vi "Monochromator API.vi"(7 "Comm":T3, 8 "error in (no error)":errorcluster, 11 "Data in out":T1={"MonoCr Port"="COM3", "Grating Selection"=enum."Grating@1", "Connection?"=TRUE, "LED Comm"=enum."LED@1", "Intensity Value"=0, "Grating Number"=1, "Wavenumber"=0, "Slit Width"=8, "Filter Num"=3, "Grating Density"=1200, "Wavelength(nm)"=400, "offset"=0.0}) -> (0 "error out":errorcluster, 2 "Connection?":bool, 3 "Data in out":T1)   [LabVIEW 2018]
uses:
  Controls/API Command.ctl
  Controls/Data highway.ctl
  Controls/LED intensity Command.ctl
  b728575c-1e5c-4404-af7d-9a6214211f88.vi
  1f586dfe-ed04-43a5-ae94-1c2b0e0186bb.vi
  98e89029-55c1-4bbe-a736-8af9f524e05c.vi
  8abd1e0c-5597-4431-9aed-95265bc6d135.vi
  59c60f5b-33d1-4c58-8755-e7aa3c9d5b29.vi
  a81fc492-f652-474c-8cd8-c09e6a443d99.vi
  8c89b708-3d56-4cfa-8980-e2557ccac631.vi
  0ff77aef-d465-45ef-9306-fcadcf69f8fd.vi
  4d5c323e-a406-4662-8192-a49ad5524d44.vi
  <vilib>/Instr/_visa.llb/VISA Configure Serial Port (Instr).vi
panel:
  in  "MonoCr Port":refnum<visa-resource-name>
  in  "Inc":bool
  out "error out":errorcluster
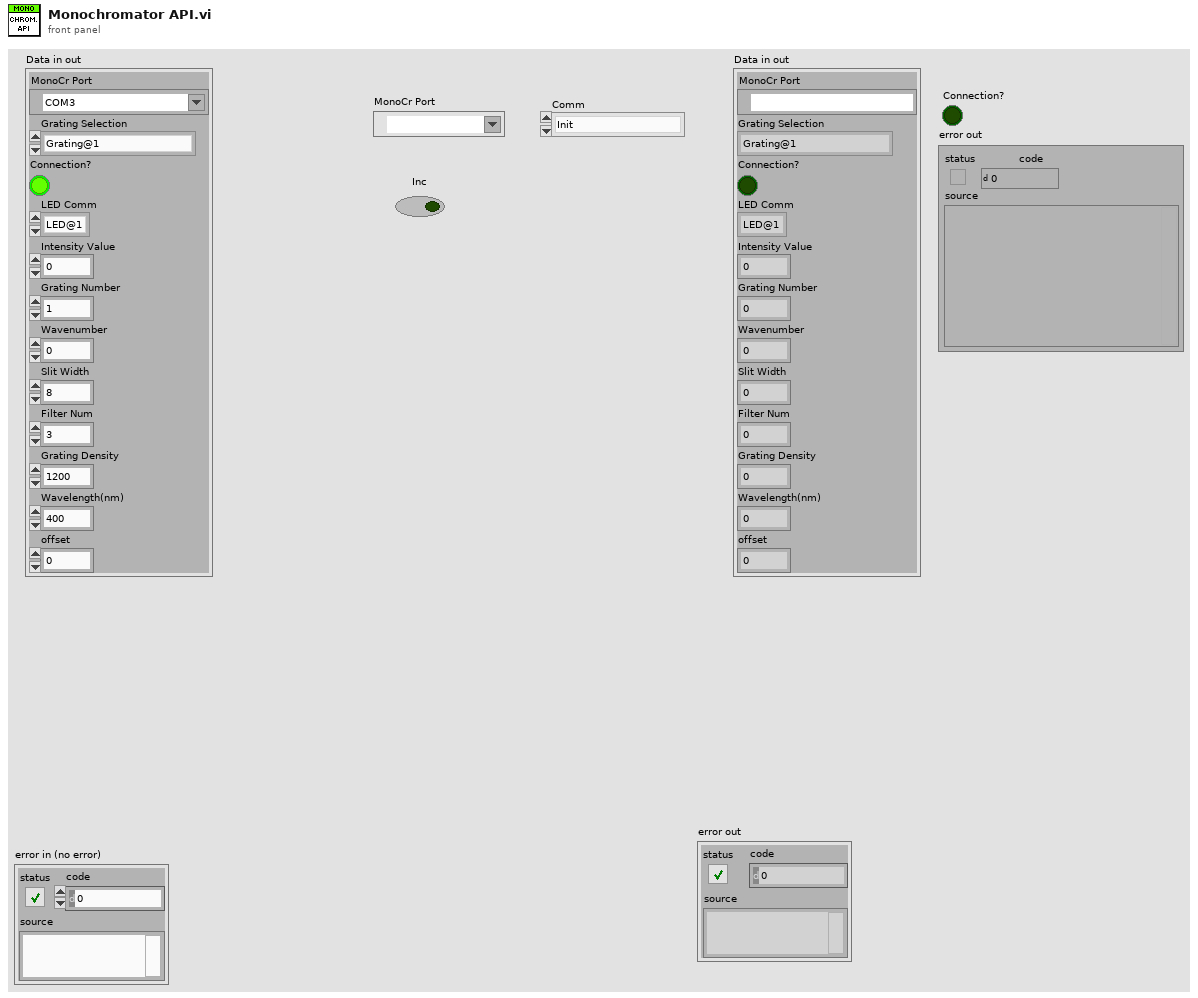
[diagram p1: front panel]
types:
  T1 = typedef "Data highway.ctl" = cluster{"MonoCr Port":refnum<visa-resource-name>, "Grating Selection":enum16{"Grating@1", "Grating@2"}, "Connection?":bool, "LED Comm":T2, "Intensity Value":i32, "Grating Number":i32, "Wavenumber":i32, "Slit Width":i32, "Filter Num":i32, "Grating Density":i32, "Wavelength(nm)":i32, "offset":dbl}
  T2 = typedef "LED intensity Command.ctl" = enum16{"LED@1", "LED@2"}
  T3 = typedef "API Command.ctl" = enum16{"Init", "Device Check", "Grating Density@1", "Grating Density@2", "SetWavelength", "Filter Selection", "Shutter open", "Shutter close", "LED Intensity", "Set Grating", "Slit Width", "Stop running", "Reset Mono", "Close"}
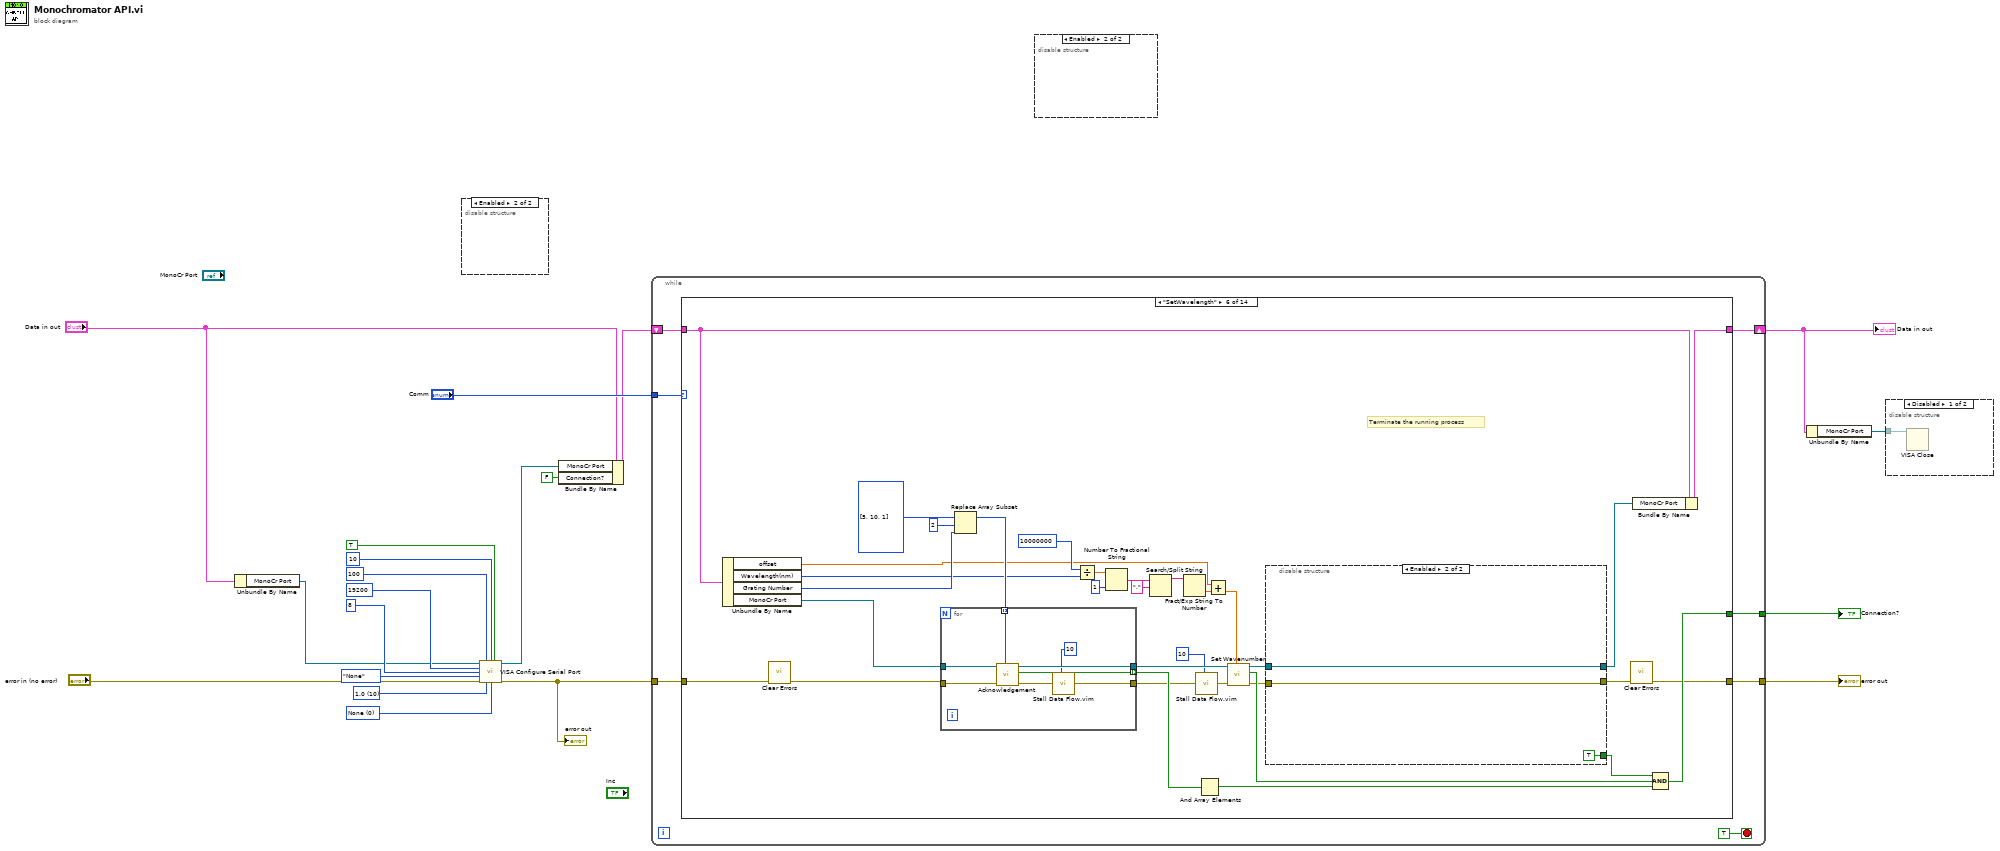
[diagram p0: block diagram]
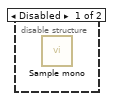
[diagram p3: hidden frame]
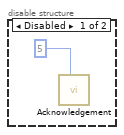
[diagram p4: hidden frame]
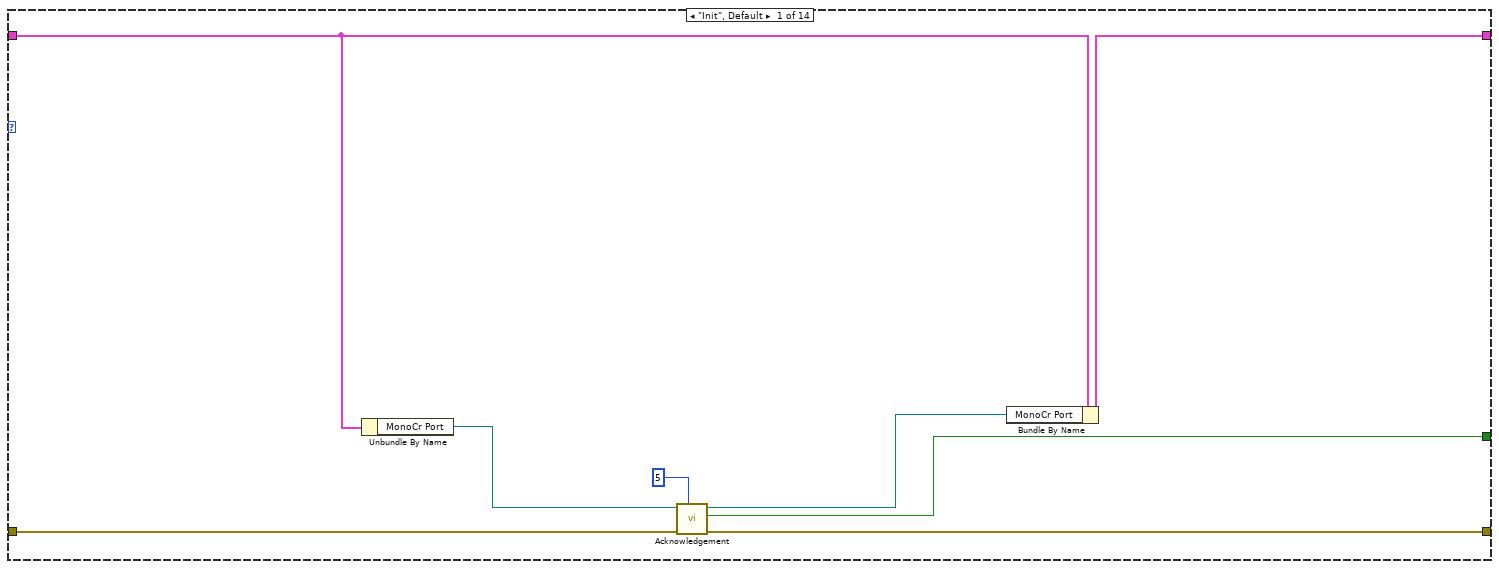
[diagram p5: hidden frame]
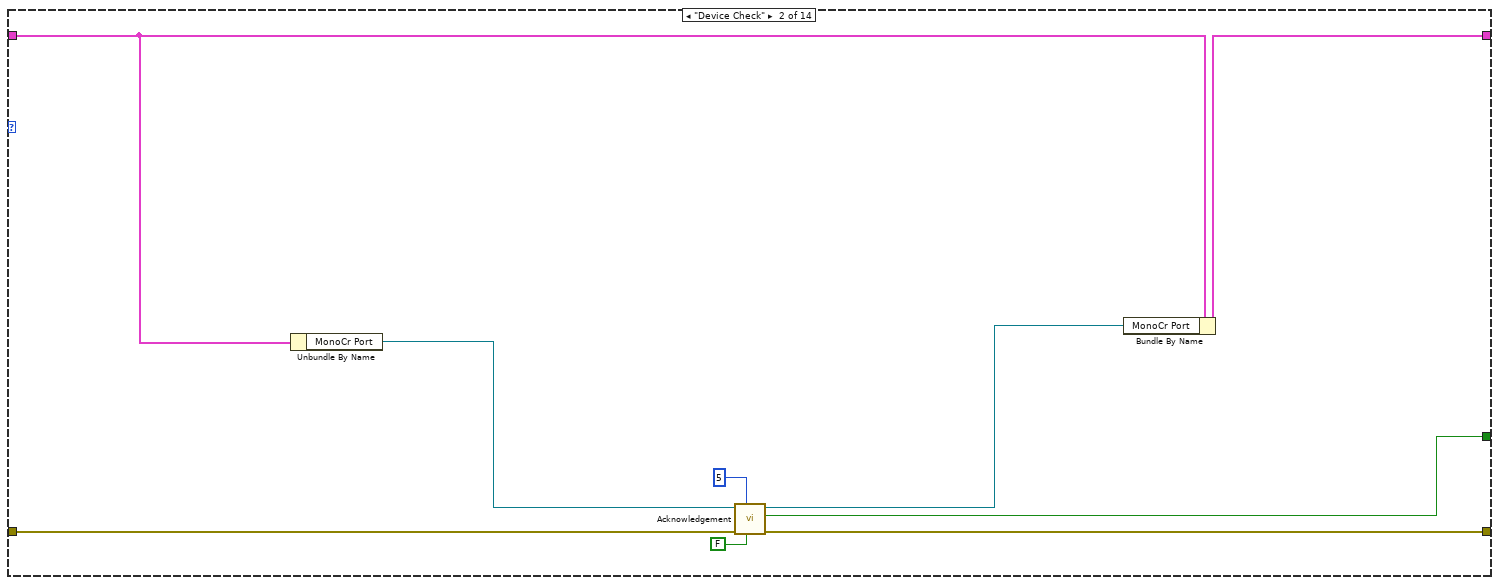
[diagram p6: hidden frame]
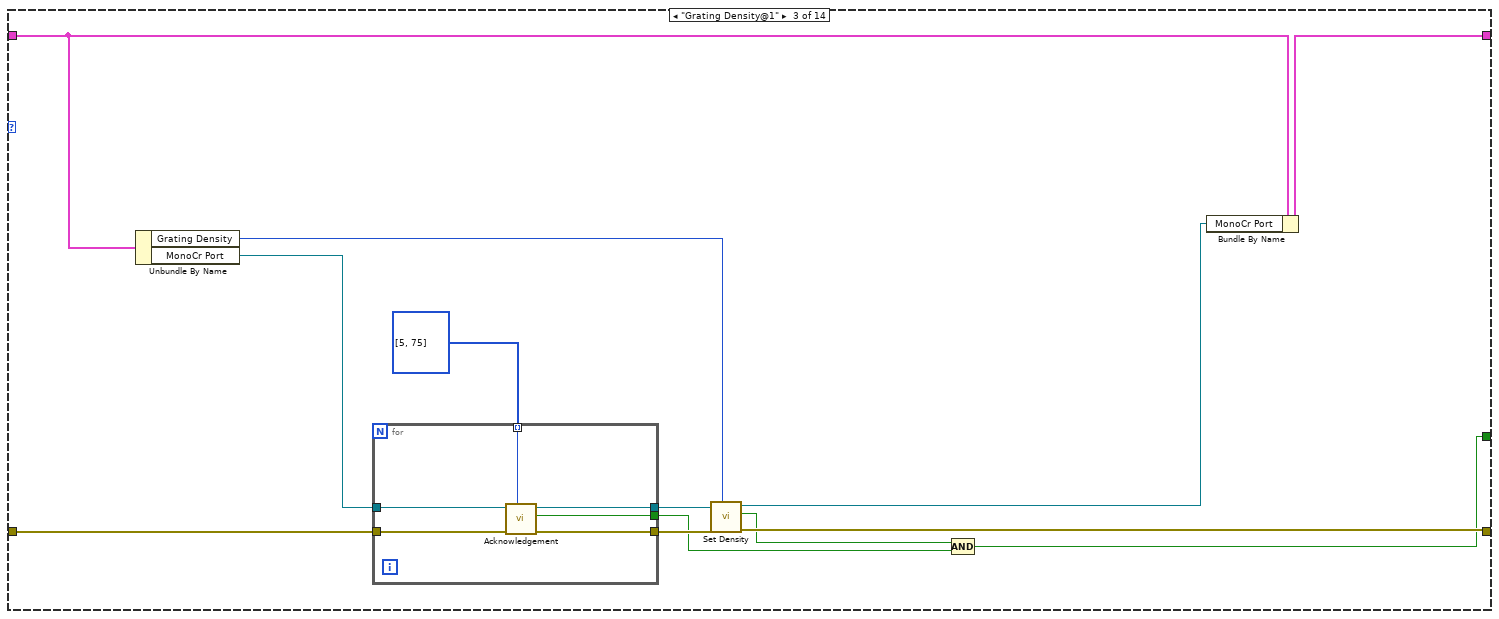
[diagram p7: hidden frame]
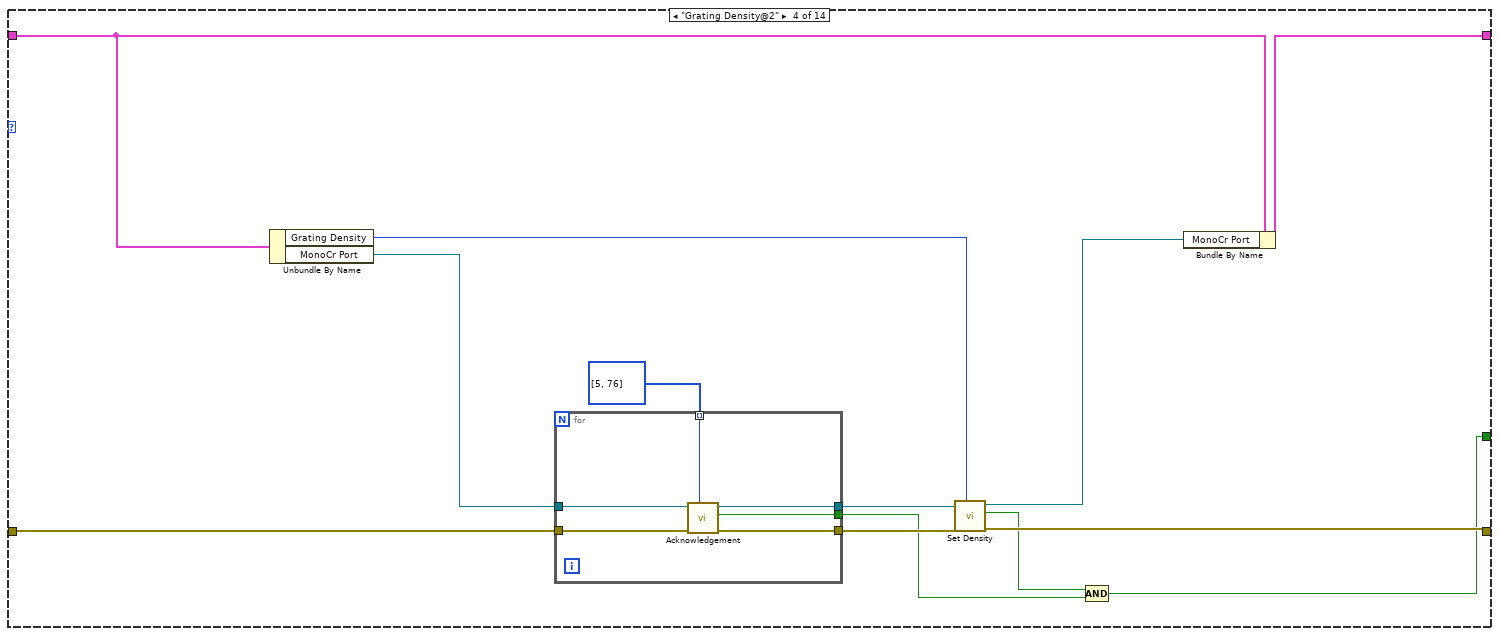
[diagram p8: hidden frame]
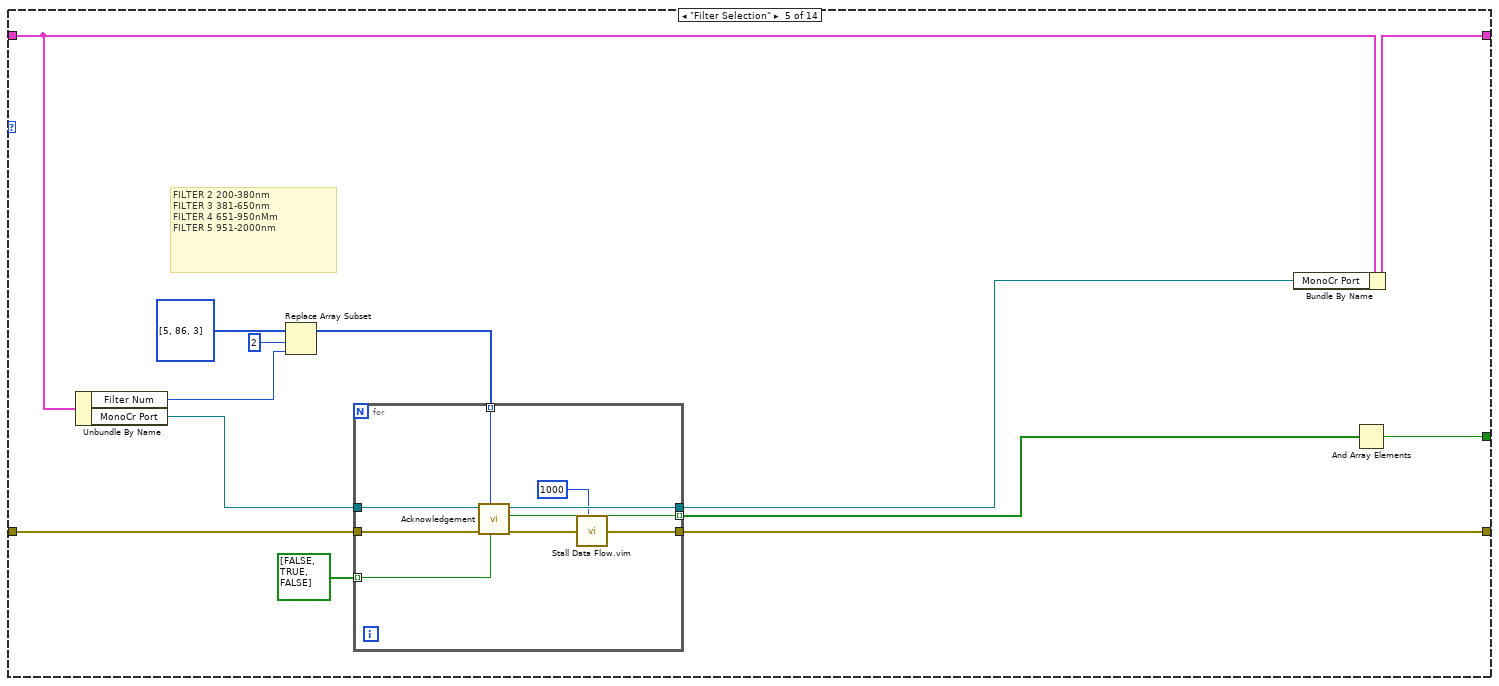
[diagram p9: hidden frame]
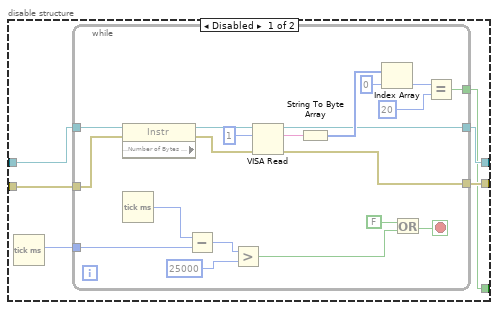
[diagram p10: hidden frame]
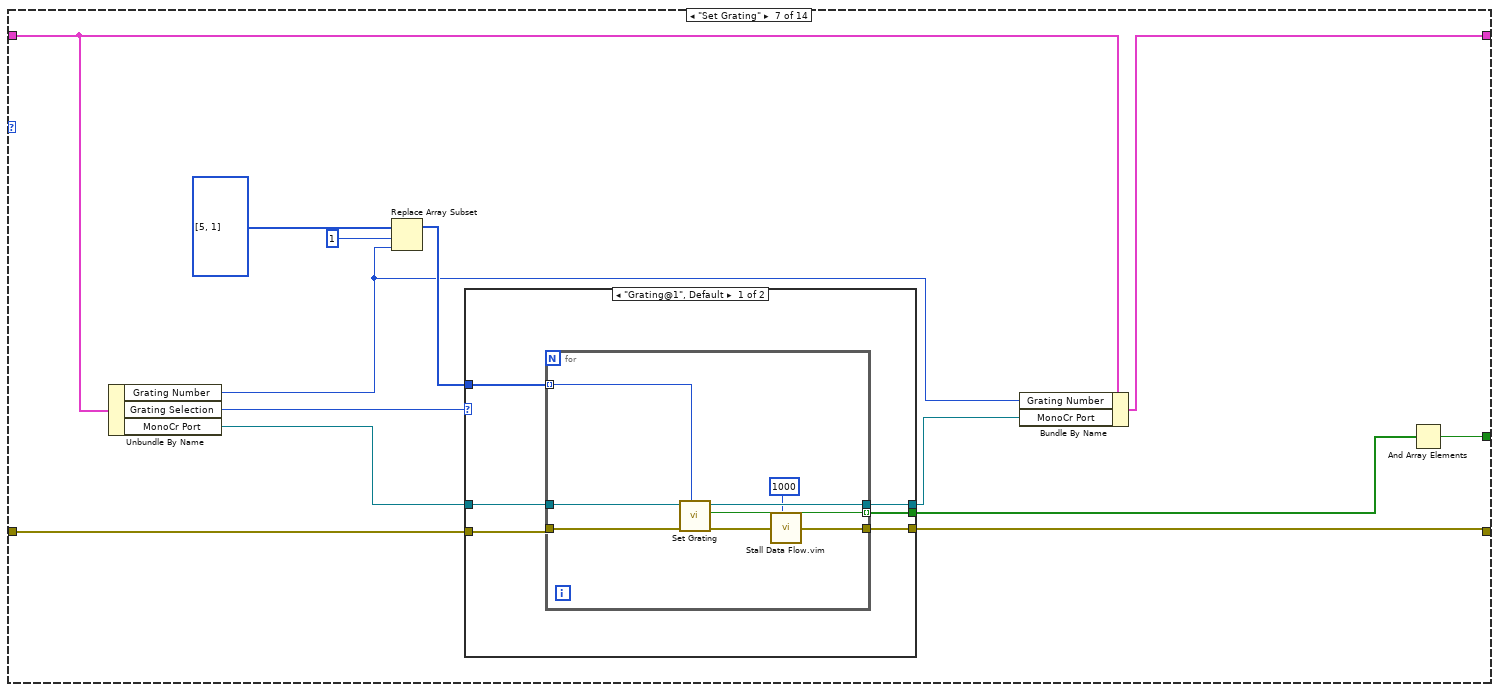
[diagram p11: hidden frame]
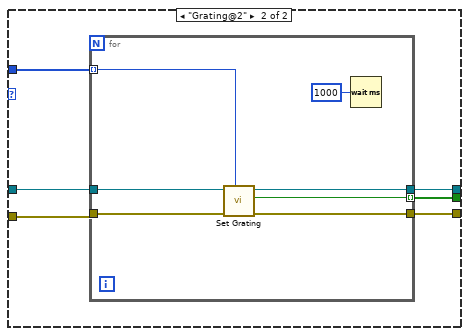
[diagram p12: hidden frame]
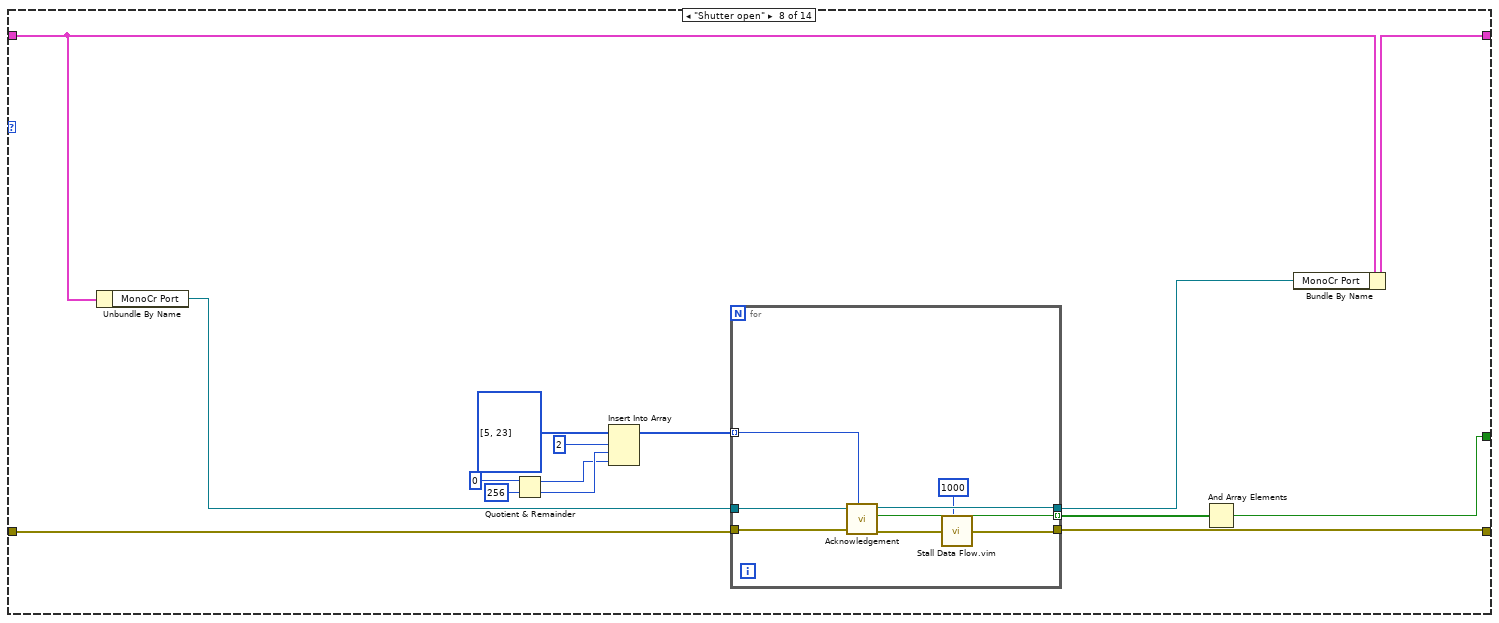
[diagram p13: hidden frame]
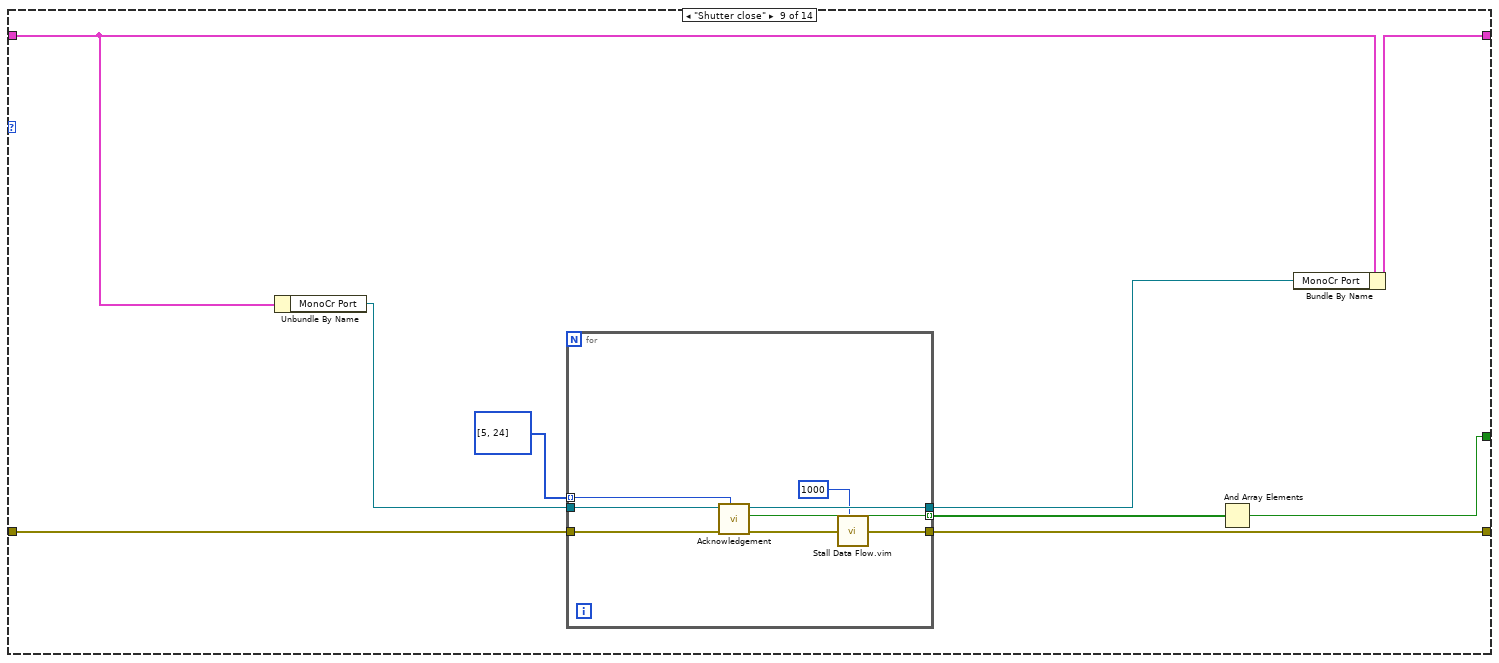
[diagram p14: hidden frame]
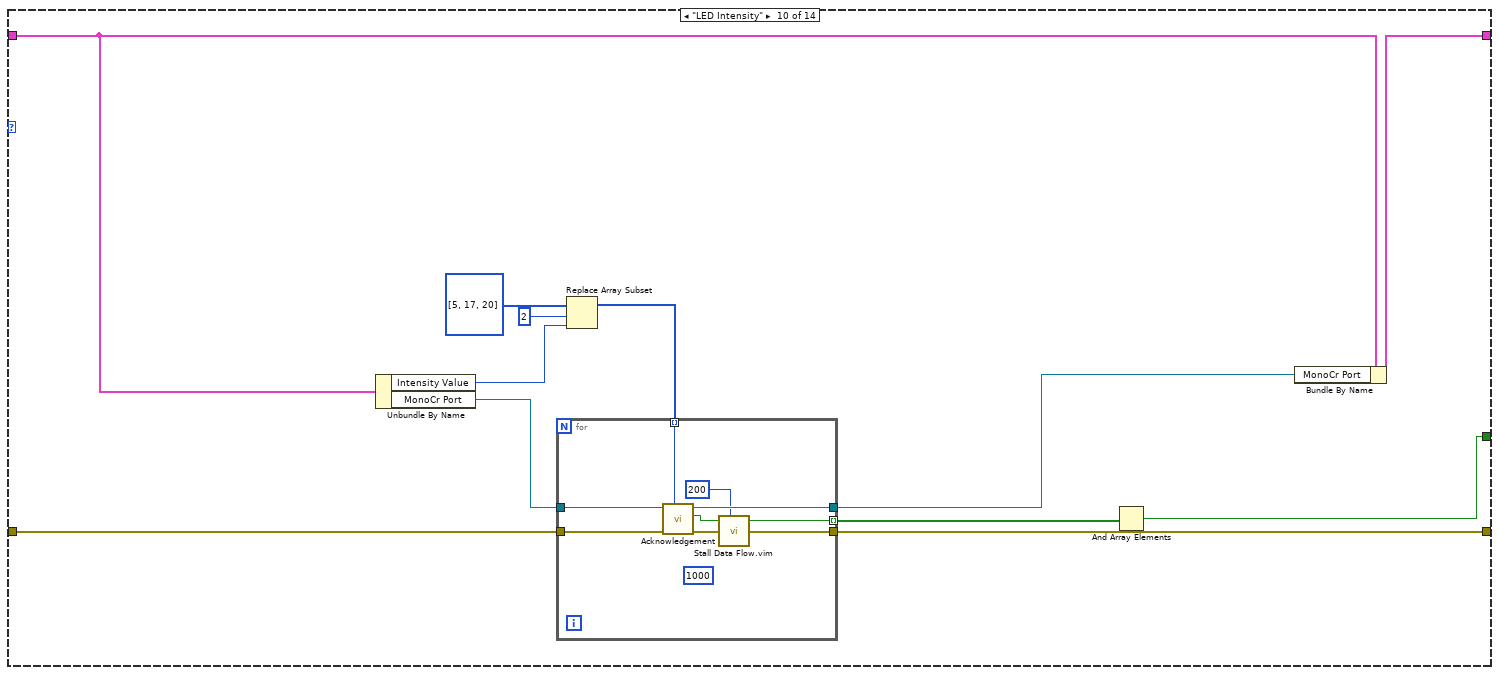
[diagram p15: hidden frame]
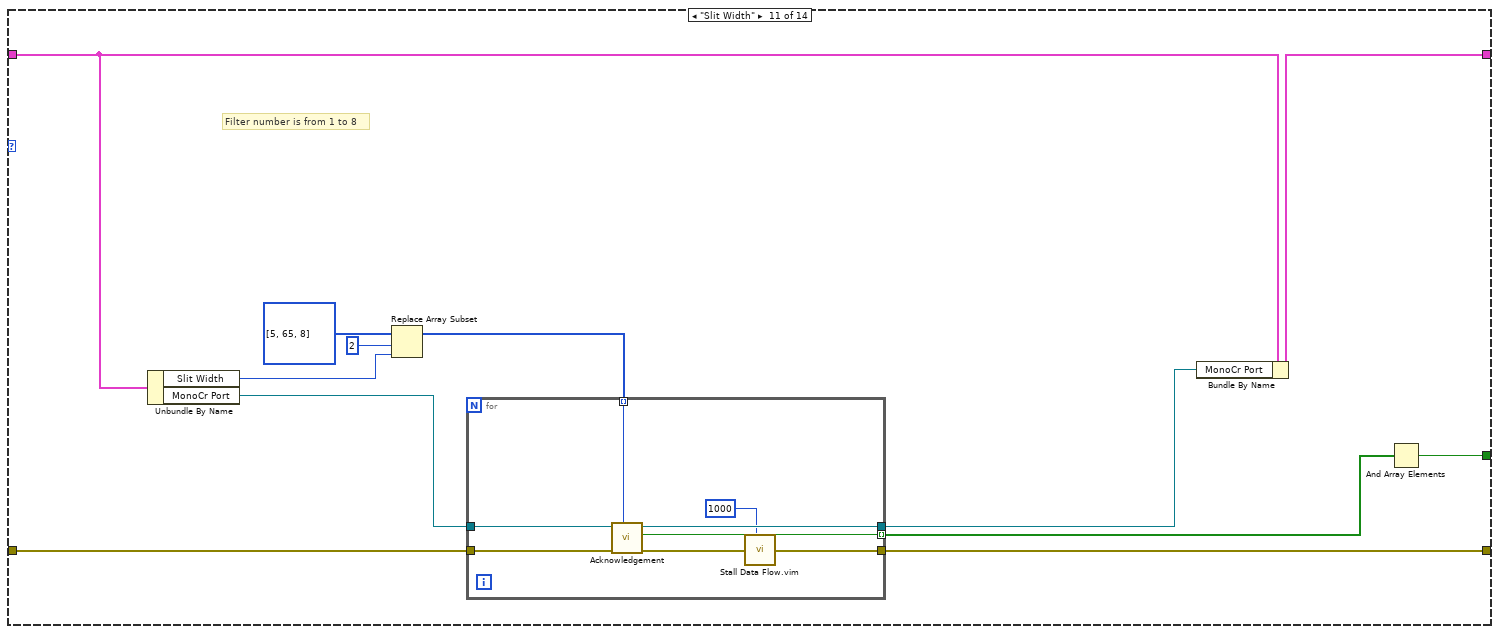
[diagram p16: hidden frame]
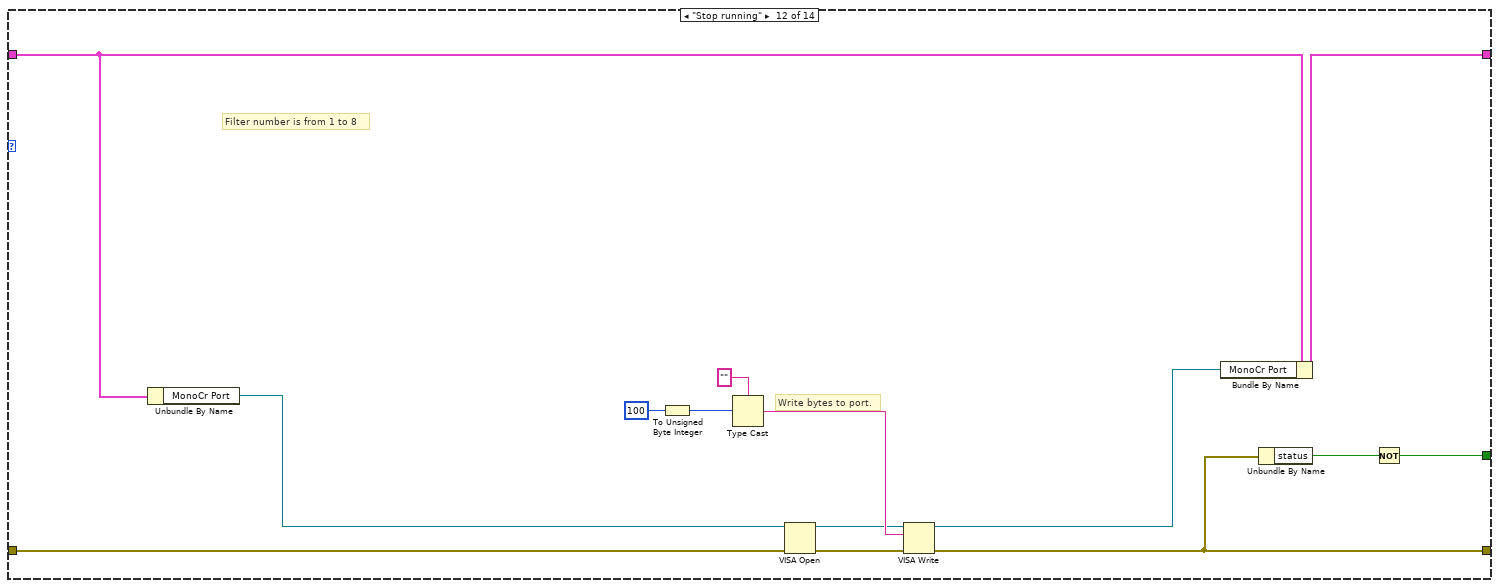
[diagram p17: hidden frame]
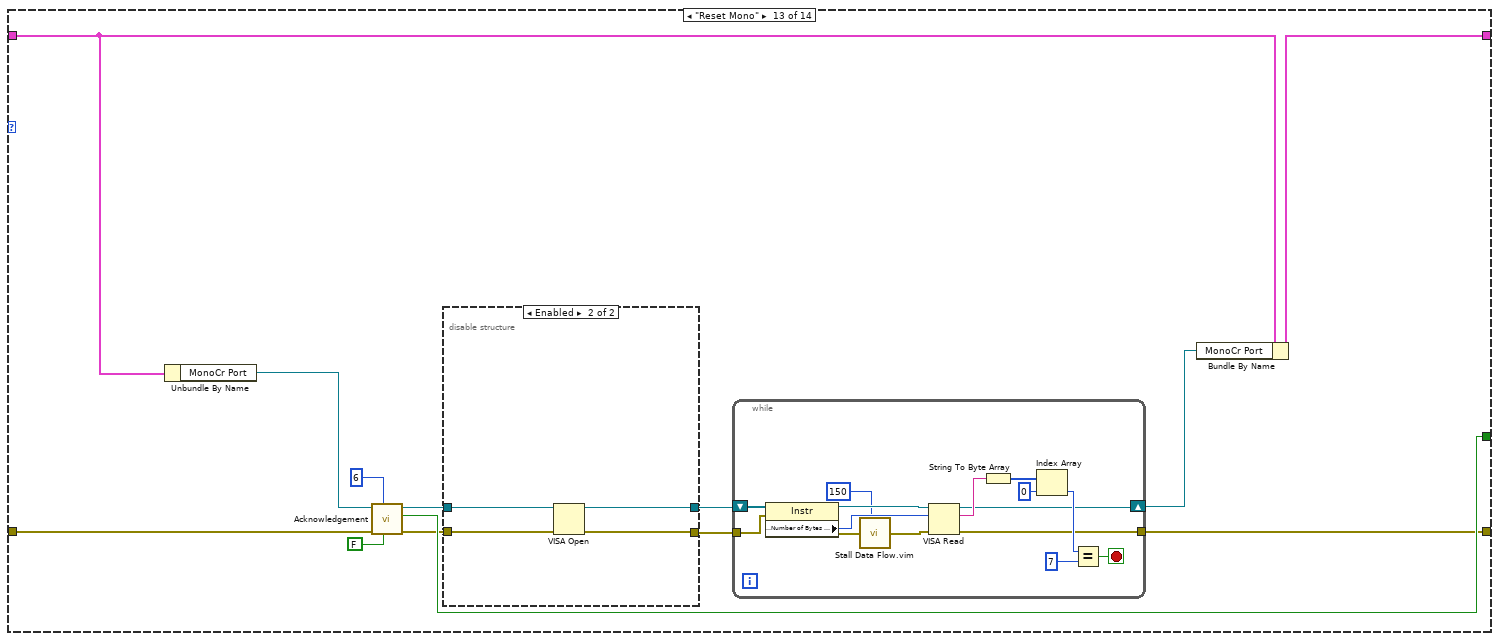
[diagram p18: hidden frame]
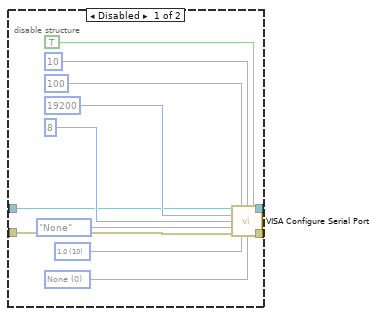
[diagram p19: hidden frame]
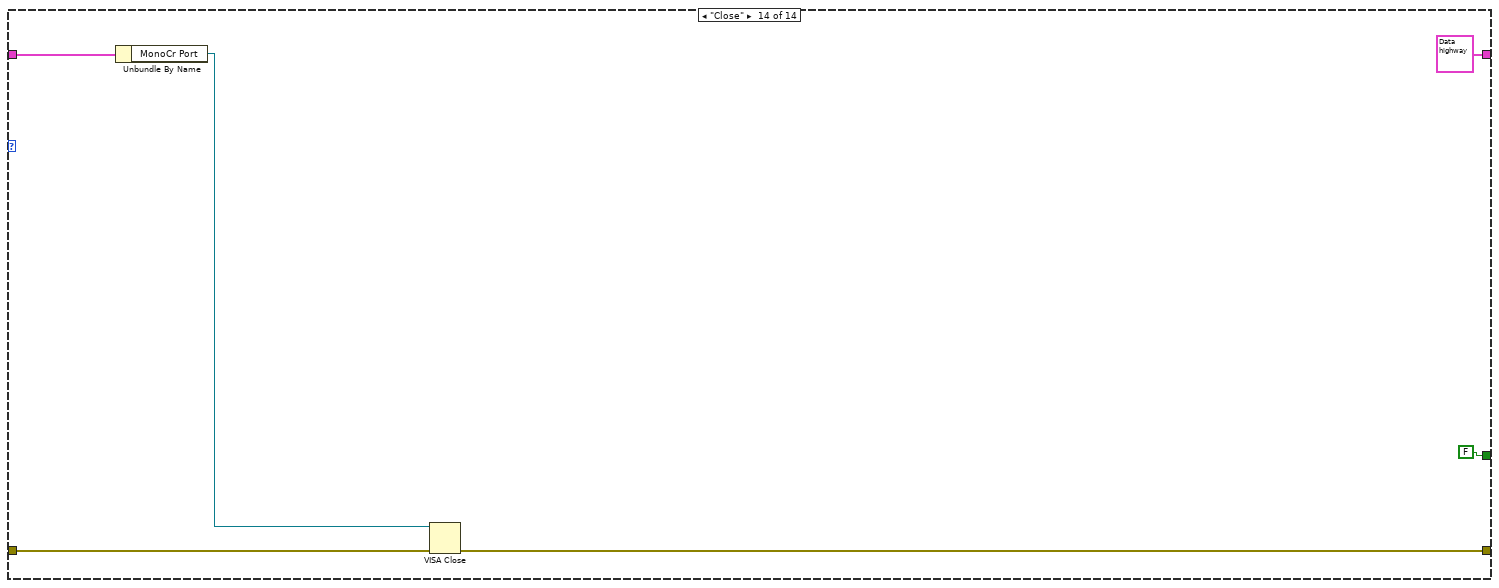
[diagram p20: hidden frame]
diagram:
  w9 = u16 0 items=["None", "XON/XOFF", "RTS/CTS", "XON/XOFF & RTS/CTS", "DTR/DSR", "XON/XOFF & DTR/DSR"] ("flow control (0:none)")
  w10 = u16 10 items=["1.0"=10, "1.5"=15, "2.0"=20] ("stop bits (10: 1 bit)")
  n1 = Unbundle By Name("Data in out") -> ("MonoCr Port"=w6:refnum<visa-resource-name>)
  n2 = disable-structure shown="Enabled" {
    frame Disabled {
      n3 = call "Acknowledgement.vi"("Numeric"=5) -> ()  [unwired: 8 in, 3 out]
    }
    frame Enabled {
    }
  }
  n4 = call-poly "VISA Configure Serial Port"("VISA resource name"=w6, "timeout (10sec)"=u32 100, "termination char\n(0xA = '\\n' = LF)"=u8 10 ("termination char\n(0xA = '\\n' = LF)"), "Enable Termination\nChar (T)"=TRUE ("Enable Termination\nChar (T)"), "baud rate (9600)"=u32 19200, "data bits (8)"=u16 8, "parity (0:none)"=enum16{"None", "Odd", "Even", "Mark", "Space"}."None", "error in (no error)"="error in (no error)", "stop bits (10: 1 bit)"=w10, "flow control (0:none)"=w9) -> ("VISA resource name out"=w7:refnum<visa-resource-name>, "error out"=w3:errorcluster)  [unwired: 4 in]
  "error out" <- w3
  n5 = Bundle By Name(cluster="Data in out", "MonoCr Port"=w7, "Connection?"=FALSE) -> (w17:T1)
  n6 = while {
    tunnel: w3 -> [w26]
    tunnel: [w25] -> w19
    tunnel: "Comm" -> [w28]
    shift-right: [w23] -> w2
    shift-left: w17 -> [w24]
    tunnel: [w22] -> w4
    stop <- TRUE stop-if-true
    n7 = case shown="\"SetWavelength\"" w28 {
      tunnel: w26 -> [w35 w45 w55 w74 w95 w138 w188 w230 w247 w265 w285 w307 w320 w357]
      tunnel: [w30 w44 w58 w77 w94 w117 w187 w226 w243 w262 w283 w298 w310 w356] -> w25
      tunnel: w24 -> [w34 w43 w57 w76 w93 w137 w186 w229 w246 w267 w287 w309 w322 w359]
      tunnel: [w32 w41 w56 w75 w91 w136 w184 w227 w244 w266 w286 w308 w321 T1 {"MonoCr Port"="", "Grating Selection"=enum."Grating@1", "Connection?"=FALSE, "LED Comm"=enum."LED@1", "Intensity Value"=0, "Grating Number"=0, "Wavenumber"=0, "Slit Width"=0, "Filter Num"=0, "Grating Density"=0, "Wavelength(nm)"=0, "offset"=0.0} ("Data in out 2")] -> w23
      tunnel: [w29 w37 w47 w66 w84 w127 w176 w222 w240 w256 w277 w296 w317 FALSE ("Connected?")] -> w22
      frame "Init", Default {
        n8 = Unbundle By Name(w34) -> ("MonoCr Port"=w33:refnum<visa-resource-name>)
        n9 = call "Acknowledgement.vi"("Numeric"=5, "error in (no error)"=w35, "VISA resource name"=w33) -> ("error out"=w30:errorcluster, "Connected?"=w29:bool, "VISA resource name out"=w31:refnum<visa-resource-name>)  [unwired: 6 in]
        n10 = Bundle By Name(cluster=w34, "MonoCr Port"=w31) -> (w32:T1)
      }
      frame "Device Check" {
        n11 = Unbundle By Name(w43) -> ("MonoCr Port"=w42:refnum<visa-resource-name>)
        n12 = call "Acknowledgement.vi"("Inc"=FALSE, "Numeric"=5, "error in (no error)"=w45, "VISA resource name"=w42) -> ("error out"=w44:errorcluster, "Connected?"=w37:bool, "VISA resource name out"=w40:refnum<visa-resource-name>)  [unwired: 5 in]
        n13 = Bundle By Name(cluster=w43, "MonoCr Port"=w40) -> (w41:T1)
      }
      frame "Grating Density@1" {
        n14 = Unbundle By Name(w57) -> ("Grating Density"=w49:i32, "MonoCr Port"=w54:refnum<visa-resource-name>)
        n15 = for {
          tunnel: [w60] -> w50
          tunnel: w54 -> [w63]
          tunnel: [w62] -> w53
          tunnel: w55 -> [w64]
          tunnel: [w61] -> w52
          tunnel: i32[] [5, 75] -> [w59] mode=indexing
          n16 = call "Acknowledgement.vi"("Numeric"=w59, "error in (no error)"=w64, "VISA resource name"=w63) -> ("error out"=w61:errorcluster, "Connected?"=w60:bool, "VISA resource name out"=w62:refnum<visa-resource-name>)  [unwired: 6 in]
        }
        n17 = call "Set Density.vi"("Density Value"=w49, "error in (no error)"=w52, "Comport"=w53) -> ("error out"=w58:errorcluster, "Set Success"=w51:bool, "Comport 2"=w48:refnum<visa-resource-name>)  [unwired: 6 in]
        n18 = Compound Arithmetic op=AND(w51, w50) -> (w47:bool)
        n19 = Bundle By Name(cluster=w57, "MonoCr Port"=w48) -> (w56:T1)
      }
      frame "Grating Density@2" {
        n20 = Unbundle By Name(w76) -> ("Grating Density"=w68:i32, "MonoCr Port"=w73:refnum<visa-resource-name>)
        n21 = for {
          tunnel: [w79] -> w69
          tunnel: w73 -> [w82]
          tunnel: [w81] -> w72
          tunnel: w74 -> [w83]
          tunnel: [w80] -> w71
          tunnel: i32[] [5, 76] -> [w78] mode=indexing
          n22 = call "Acknowledgement.vi"("Numeric"=w78, "error in (no error)"=w83, "VISA resource name"=w82) -> ("error out"=w80:errorcluster, "Connected?"=w79:bool, "VISA resource name out"=w81:refnum<visa-resource-name>)  [unwired: 6 in]
        }
        n23 = call "Set Density.vi"("Density Value"=w68, "error in (no error)"=w71, "Comport"=w72) -> ("error out"=w77:errorcluster, "Set Success"=w70:bool, "Comport 2"=w67:refnum<visa-resource-name>)  [unwired: 6 in]
        n24 = Compound Arithmetic op=AND(w70, w69) -> (w66:bool)
        n25 = Bundle By Name(cluster=w76, "MonoCr Port"=w67) -> (w75:T1)
      }
      frame "Filter Selection" {
        # "FILTER 2 200-380nm\nFILTER 3 381-650nm\nFILTER 4 651-950nMm\nFILTER 5 951-2000nm"
        n26 = Unbundle By Name(w93) -> ("Filter Num"=w87:i32, "MonoCr Port"=w92:refnum<visa-resource-name>)
        n27 = Replace Array Subset(array=i32[] [5, 86, 3] ("Numeric"), new element=w87, index=2) -> (w89:i32[])
        n28 = for {
          tunnel: w89 -> [w105] mode=indexing
          tunnel: [w100] -> w90 mode=indexing
          tunnel: w92 -> [w101]
          tunnel: [w102] -> w85
          tunnel: w95 -> [w104]
          tunnel: [w98] -> w94
          tunnel: bool[] [FALSE, TRUE, FALSE] ("Inc") -> [w99] mode=indexing
          n29 = call "Acknowledgement.vi"("Inc"=w99, "Numeric"=w105, "error in (no error)"=w104, "VISA resource name"=w101) -> ("error out"=w103:errorcluster, "Connected?"=w100:bool, "VISA resource name out"=w102:refnum<visa-resource-name>)  [unwired: 5 in]
          n30 = call "Stall Data Flow.vim"("value in"=w103, "milliseconds to wait"=u32 1000) -> ("value out"=w98:errorcluster)  [unwired: 1 out]
        }
        n31 = Bundle By Name(cluster=w93, "MonoCr Port"=w85) -> (w91:T1)
        n32 = And Array Elements(Boolean array=w90) -> (logical AND=w84:bool)
      }
      frame "SetWavelength" {
        # "Terminate the running process"
        n33 = Unbundle By Name(w137) -> ("offset"=w106:dbl, "Wavelength(nm)"=w116:i32, "Grating Number"=w128:i32, "MonoCr Port"=w134:refnum<visa-resource-name>)
        n34 = call <vilib>:"Clear Errors.vi"("error in (no error)"=w138) -> ("error out"=w135:errorcluster)  [unwired: 5 in, 1 out]
        n35 = Replace Array Subset(array=i32[] [5, 10, 1] ("Numeric"), new element=w128, index=2 ("new element/subarray")) -> (w130:i32[])
        n36 = for {
          tunnel: [w171] -> w132 mode=indexing
          tunnel: w135 -> [w175]
          tunnel: [w169] -> w121
          tunnel: w134 -> [w173]
          tunnel: [w172] -> w122
          tunnel: w130 -> [w170] mode=indexing
          n37 = call "Acknowledgement.vi"("Numeric"=w170, "error in (no error)"=w175, "VISA resource name"=w173) -> ("error out"=w174:errorcluster, "Connected?"=w171:bool, "VISA resource name out"=w172:refnum<visa-resource-name>)  [unwired: 6 in]
          n38 = call "Stall Data Flow.vim"("value in"=w174, "milliseconds to wait"=u32 10) -> ("value out"=w169:errorcluster)  [unwired: 1 out]
        }
        n39 = Divide(x=10000000, y=w116) -> (x/y=w113:dbl)
        n40 = Number To Fractional String(number=w113, precision (6)=i16 1) -> (F-format string=w111:string)  [unwired: 2 in]
        n41 = Search/Split String(string=w111, search string/char (-)=".") -> (substring before match=w109:string)  [unwired: 1 in, 2 out]
        n42 = Fract/Exp String To Number(string=w109) -> (number=w108:dbl)  [unwired: 3 in, 1 out]
        n43 = call "Stall Data Flow.vim"("value in"=w121, "milliseconds to wait"=u32 10) -> ("value out"=w120:errorcluster)  [unwired: 1 out]
        n44 = And Array Elements(Boolean array=w132) -> (logical AND=w129:bool)
        n45 = Add(x=w106, y=w108) -> (x+y=w107:dbl)
        n46 = call "Set Wavenumber.vi"("Wave number"=w107, "error in (no error)"=w120, "Comport"=w122) -> ("error out"=w125:errorcluster, "Set Success"=w133:bool, "Comport 2"=w126:refnum<visa-resource-name>)  [unwired: 6 in]
        n47 = disable-structure shown="Enabled" {
          disable-tunnel: w126 -> [w144 w167]
          disable-tunnel: w125 -> [w143 w166]
          disable-tunnel: [w142 w167] -> w124
          disable-tunnel: [w141 w166] -> w118
          disable-tunnel: [w139 TRUE] -> w114
          frame Disabled {
            n48 = Tick Count (ms)() -> (millisecond timer value=w140:u32)
            n49 = while {
              tunnel: w143 -> [w156]
              tunnel: [w154] -> w141
              tunnel: w144 -> [w157]
              tunnel: [w155] -> w142
              tunnel: w140 -> [w152]
              tunnel: [w146] -> w139
              stop <- w149 stop-if-true
              n50 = property class="Instr" props=["Serial Settings:Number of Bytes at Serial Port"](reference=w157, error in=w156) -> (reference out=w163:refnum<visa-resource-name>, error out=w164:errorcluster)  [unwired: 1 out]
              n51 = Tick Count (ms)() -> (millisecond timer value=w153:u32)
              n52 = Subtract(x=w153, y=w152) -> (x-y=w151:u32)
              n53 = Greater?(x=w151, y=u32 25000) -> (0:w148:bool)
              n54 = VISA Read(VISA resource name=w163, byte count=u32 1, error in (no error)=w164) -> (VISA resource name out=w155:refnum<visa-resource-name>, read buffer=w160:string, error out=w154:errorcluster)  [unwired: 1 out]
              n55 = String To Byte Array(string=w160) -> (unsigned byte array=w161:u8[])
              n56 = Index Array(array=w161, index=0) -> (element=w162:u8)
              n57 = Or(x=FALSE, y=w148) -> (x .or. y?=w149:bool)
              n58 = Equal?(x=w162, y=u8 20) -> (x = y?=w146:bool)
            }
          }
          frame Enabled {
          }
        }
        n59 = call <vilib>:"Clear Errors.vi"("error in (no error)"=w118) -> ("error out"=w117:errorcluster)  [unwired: 5 in, 1 out]
        n60 = Bundle By Name(cluster=w137, "MonoCr Port"=w124) -> (w136:T1)
        n61 = Compound Arithmetic op=AND(w114, w133, w129) -> (w127:bool)
      }
      frame "Set Grating" {
        n62 = Unbundle By Name(w186) -> ("Grating Number"=w178:i32, "Grating Selection"=w183:enum16{"Grating@1", "Grating@2"}, "MonoCr Port"=w185:refnum<visa-resource-name>)
        n63 = Replace Array Subset(array=i32[] [5, 1], new element=w178, index=1 ("new element/subarray")) -> (w180:i32[])
        n64 = case shown="\"Grating@1\", Default" w183 {
          tunnel: w188 -> [w194 w208]
          tunnel: [w193 w207] -> w187
          tunnel: w185 -> [w192 w206]
          tunnel: [w191 w205] -> w177
          tunnel: [w190 w204] -> w181
          tunnel: w180 -> [w189 w203]
          frame "Grating@1", Default {
            n65 = for {
              tunnel: [w198] -> w190 mode=indexing
              tunnel: w194 -> [w202]
              tunnel: [w196] -> w193
              tunnel: w192 -> [w200]
              tunnel: [w199] -> w191
              tunnel: w189 -> [w197] mode=indexing
              n66 = call "Set Grating.vi"("Numeric"=w197, "error in (no error)"=w202, "VISA resource name"=w200) -> ("error out"=w201:errorcluster, "Connected? 2"=w198:bool, "VISA resource name out"=w199:refnum<visa-resource-name>)  [unwired: 6 in]
              n67 = call "Stall Data Flow.vim"("value in"=w201, "milliseconds to wait"=u32 1000) -> ("value out"=w196:errorcluster)  [unwired: 1 out]
            }
          }
          frame "Grating@2" {
            n68 = for {
              tunnel: [w211] -> w204 mode=indexing
              tunnel: w208 -> [w215]
              tunnel: [w214] -> w207
              tunnel: w206 -> [w213]
              tunnel: [w212] -> w205
              tunnel: w203 -> [w209] mode=indexing
              n69 = call "Set Grating.vi"("Numeric"=w209, "error in (no error)"=w215, "VISA resource name"=w213) -> ("error out"=w214:errorcluster, "Connected? 2"=w211:bool, "VISA resource name out"=w212:refnum<visa-resource-name>)  [unwired: 6 in]
              n70 = Wait (ms)(milliseconds to wait=u32 1000) -> ()  [unwired: 1 out]
            }
          }
        }
        n71 = Bundle By Name(cluster=w186, "Grating Number"=w178, "MonoCr Port"=w177) -> (w184:T1)
        n72 = And Array Elements(Boolean array=w181) -> (logical AND=w176:bool)
      }
      frame "Shutter open" {
        n73 = Unbundle By Name(w229) -> ("MonoCr Port"=w228:refnum<visa-resource-name>)
        n74 = Quotient & Remainder(x=u32 0, y=u32 256) -> (x-y*floor(x/y)=w216:u32, floor(x/y)=w217:u32)
        n75 = Insert Into Array(array=i32[] [5, 23] ("Numeric"), index=2, new element #1=w217, new element #2=w216) -> (w219:i32[])
        n76 = for {
          tunnel: w228 -> [w237]
          tunnel: [w235] -> w223
          tunnel: w230 -> [w238]
          tunnel: [w232] -> w226
          tunnel: w219 -> [w234] mode=indexing
          tunnel: [w233] -> w224 mode=indexing
          n77 = call "Acknowledgement.vi"("Numeric"=w234, "error in (no error)"=w238, "VISA resource name"=w237) -> ("error out"=w236:errorcluster, "Connected?"=w233:bool, "VISA resource name out"=w235:refnum<visa-resource-name>)  [unwired: 6 in]
          n78 = call "Stall Data Flow.vim"("value in"=w236, "milliseconds to wait"=u32 1000) -> ("value out"=w232:errorcluster)  [unwired: 1 out]
        }
        n79 = And Array Elements(Boolean array=w224) -> (logical AND=w222:bool)
        n80 = Bundle By Name(cluster=w229, "MonoCr Port"=w223) -> (w227:T1)
      }
      frame "Shutter close" {
        n81 = Unbundle By Name(w246) -> ("MonoCr Port"=w245:refnum<visa-resource-name>)
        n82 = for {
          tunnel: [w251] -> w242 mode=indexing
          tunnel: w247 -> [w255]
          tunnel: [w249] -> w243
          tunnel: w245 -> [w254]
          tunnel: [w252] -> w241
          tunnel: i32[] [5, 24] ("Numeric") -> [w250] mode=indexing
          n83 = call "Acknowledgement.vi"("Numeric"=w250, "error in (no error)"=w255, "VISA resource name"=w254) -> ("error out"=w253:errorcluster, "Connected?"=w251:bool, "VISA resource name out"=w252:refnum<visa-resource-name>)  [unwired: 6 in]
          n84 = call "Stall Data Flow.vim"("value in"=w253, "milliseconds to wait"=u32 1000) -> ("value out"=w249:errorcluster)  [unwired: 1 out]
        }
        n85 = And Array Elements(Boolean array=w242) -> (logical AND=w240:bool)
        n86 = Bundle By Name(cluster=w246, "MonoCr Port"=w241) -> (w244:T1)
      }
      frame "LED Intensity" {
        n87 = Unbundle By Name(w267) -> ("Intensity Value"=w258:i32, "MonoCr Port"=w264:refnum<visa-resource-name>)
        n88 = Replace Array Subset(array=i32[] [5, 17, 20] ("Numeric"), new element=w258, index=2) -> (w260:i32[])
        n89 = for {
          tunnel: [w271] -> w261 mode=indexing
          tunnel: w260 -> [w270] mode=indexing
          tunnel: w264 -> [w273]
          tunnel: [w272] -> w257
          tunnel: w265 -> [w275]
          tunnel: [w269] -> w262
          (unwired) u32 1000 ("milliseconds to wait")
          n90 = call "Acknowledgement.vi"("Numeric"=w270, "error in (no error)"=w275, "VISA resource name"=w273) -> ("error out"=w274:errorcluster, "Connected?"=w271:bool, "VISA resource name out"=w272:refnum<visa-resource-name>)  [unwired: 6 in]
          n91 = call "Stall Data Flow.vim"("value in"=w274, "milliseconds to wait"=u32 200) -> ("value out"=w269:errorcluster)  [unwired: 1 out]
        }
        n92 = And Array Elements(Boolean array=w261) -> (logical AND=w256:bool)
        n93 = Bundle By Name(cluster=w267, "MonoCr Port"=w257) -> (w266:T1)
      }
      frame "Slit Width" {
        # "Filter number is from 1 to 8"
        n94 = Unbundle By Name(w287) -> ("Slit Width"=w280:i32, "MonoCr Port"=w284:refnum<visa-resource-name>)
        n95 = Replace Array Subset(array=i32[] [5, 65, 8] ("Numeric"), new element=w280, index=2) -> (w281:i32[])
        n96 = for {
          tunnel: w284 -> [w294]
          tunnel: [w292] -> w278
          tunnel: w285 -> [w295]
          tunnel: [w289] -> w283
          tunnel: w281 -> [w291] mode=indexing
          tunnel: [w290] -> w279 mode=indexing
          n97 = call "Acknowledgement.vi"("Numeric"=w291, "error in (no error)"=w295, "VISA resource name"=w294) -> ("error out"=w293:errorcluster, "Connected?"=w290:bool, "VISA resource name out"=w292:refnum<visa-resource-name>)  [unwired: 6 in]
          n98 = call "Stall Data Flow.vim"("value in"=w293, "milliseconds to wait"=u32 1000) -> ("value out"=w289:errorcluster)  [unwired: 1 out]
        }
        n99 = Bundle By Name(cluster=w287, "MonoCr Port"=w278) -> (w286:T1)
        n100 = And Array Elements(Boolean array=w279) -> (logical AND=w277:bool)
      }
      frame "Stop running" {
        # "Write bytes to port."
        # "Filter number is from 1 to 8"
        n101 = Unbundle By Name(w309) -> ("MonoCr Port"=w305:refnum<visa-resource-name>)
        n102 = To Unsigned Byte Integer(number=u8 100) -> (unsigned 8bit integer=w300:u8)
        n103 = Type Cast(type="", x=w300) -> (*(type *) &x=w304:string)
        n104 = VISA Open(error in (no error)=w307, VISA resource name=w305) -> (VISA resource name=w303:refnum<visa-resource-name>, error out=w302:errorcluster)  [unwired: 3 in]
        n105 = VISA Write(VISA resource name=w303, write buffer=w304, error in (no error)=w302) -> (VISA resource name out=w306:refnum<visa-resource-name>, error out=w298:errorcluster)  [unwired: 1 out]
        n106 = Bundle By Name(cluster=w309, "MonoCr Port"=w306) -> (w308:T1)
        n107 = Unbundle By Name(w298) -> ("status"=w297:bool)
        n108 = Not(x=w297) -> (.not. x?=w296:bool)
      }
      frame "Reset Mono" {
        n109 = Unbundle By Name(w322) -> ("MonoCr Port"=w319:refnum<visa-resource-name>)
        n110 = call "Acknowledgement.vi"("Inc"=FALSE, "Numeric"=6, "error in (no error)"=w320, "VISA resource name"=w319) -> ("error out"=w312:errorcluster, "Connected?"=w317:bool, "VISA resource name out"=w314:refnum<visa-resource-name>)  [unwired: 5 in]
        n111 = disable-structure shown="Enabled" {
          disable-tunnel: w314 -> [w326 w338]
          disable-tunnel: [w325 w335] -> w313
          disable-tunnel: w312 -> [w324 w337]
          disable-tunnel: [w323 w336] -> w311
          frame Disabled {
            w334 = u16 0 items=["None", "XON/XOFF", "RTS/CTS", "XON/XOFF & RTS/CTS", "DTR/DSR", "XON/XOFF & DTR/DSR"] ("flow control (0:none)")
            w333 = u16 10 items=["1.0"=10, "1.5"=15, "2.0"=20] ("stop bits (10: 1 bit)")
            n112 = call-poly "VISA Configure Serial Port"("VISA resource name"=w326, "timeout (10sec)"=u32 100, "termination char\n(0xA = '\\n' = LF)"=u8 10 ("termination char\n(0xA = '\\n' = LF)"), "Enable Termination\nChar (T)"=TRUE ("Enable Termination\nChar (T)"), "baud rate (9600)"=u32 19200, "data bits (8)"=u16 8, "parity (0:none)"=enum16{"None", "Odd", "Even", "Mark", "Space"}."None", "error in (no error)"=w324, "stop bits (10: 1 bit)"=w333, "flow control (0:none)"=w334) -> ("VISA resource name out"=w325:refnum<visa-resource-name>, "error out"=w323:errorcluster)  [unwired: 4 in]
          }
          frame Enabled {
            n113 = VISA Open(error in (no error)=w337, VISA resource name=w338) -> (VISA resource name=w335:refnum<visa-resource-name>, error out=w336:errorcluster)  [unwired: 3 in]
          }
        }
        n114 = while {
          tunnel: w311 -> [w344]
          shift-right: [w342] -> w315
          shift-left: w313 -> [w345]
          tunnel: [w341] -> w310
          stop <- w343 stop-if-true
          n115 = property class="Instr"(reference=w345, error in=w344) -> (reference out=w351:refnum<visa-resource-name>, error out=w352:errorcluster, "Serial Settings:Number of Bytes at Serial Port"=w353:u32)
          n116 = call "Stall Data Flow.vim"("value in"=w352, "milliseconds to wait"=u32 150) -> ("value out"=w340:errorcluster)  [unwired: 1 out]
          n117 = VISA Read(VISA resource name=w351, byte count=w353, error in (no error)=w340) -> (VISA resource name out=w342:refnum<visa-resource-name>, read buffer=w348:string, error out=w341:errorcluster)  [unwired: 1 out]
          n118 = String To Byte Array(string=w348) -> (unsigned byte array=w349:u8[])
          n119 = Index Array(array=w349, index=0) -> (element=w350:u8)
          n120 = Equal?(x=w350, y=u8 7) -> (x = y?=w343:bool)
        }
        n121 = Bundle By Name(cluster=w322, "MonoCr Port"=w315) -> (w321:T1)
      }
      frame "Close" {
        n122 = Unbundle By Name(w359) -> ("MonoCr Port"=w358:refnum<visa-resource-name>)
        n123 = VISA Close(VISA resource name=w358, error in (no error)=w357) -> (error out=w356:errorcluster)
      }
    }
  }
  "error out" <- w19
  "Data in out" <- w2
  "Connection?" <- w4
  n124 = disable-structure shown="Enabled" {
    frame Disabled {
      n125 = call "Sample mono.vi"() -> ()  [unwired: 12 in]
    }
    frame Enabled {
    }
  }
  n126 = Unbundle By Name(w2) -> ("MonoCr Port"=w1:refnum<visa-resource-name>)
  n127 = disable-structure shown="Disabled" {
    disable-tunnel: w1 -> [w360 _]
    frame Disabled {
      n128 = VISA Close(VISA resource name=w360) -> ()  [unwired: 1 in, 1 out]
    }
    frame Enabled {
    }
  }
